vi "test Get Array Size.vi"(8 "error in (no error)":errorcluster, 11 "TestCase in":refnum<class "Python String Parsing Utility Tests.lvclass">) -> (0 "error out":errorcluster, 3 "TestCase out":refnum<class "Python String Parsing Utility Tests.lvclass">)   [LabVIEW 2020, in "Python String Parsing Utility Tests.lvclass"]
uses:
  Python String Parsing Utility Tests.lvclass
  Python String Parsing Utility Tests.lvclass/Python String Parsing Utility Tests.ctl
  <vilib>/addons/_JKI Toolkits/VI Tester/TestCase.llb/TestCase.lvclass
  source/jki_python_data_tools.lvlib
  C:/Program Files/National Instruments/LabVIEW 2020/vi.lib/addons/_JKI Toolkits/VI Tester/TestCase.llb/TestCase.lvclass
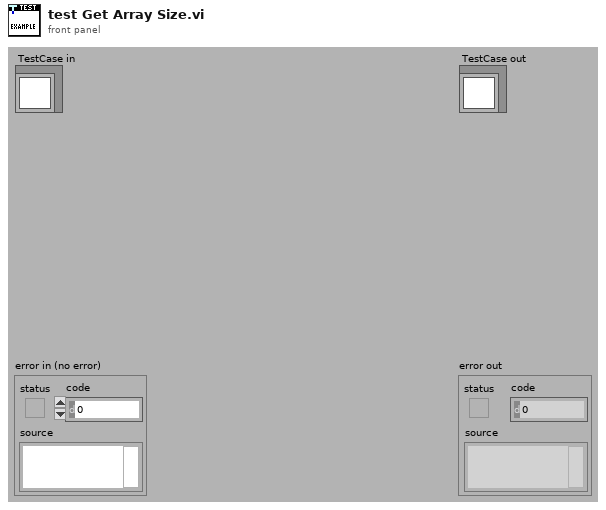
[diagram p1: front panel]
types:
  T1 = cluster{"Input":string, "Expected Result":i32, "Comment":string}[]
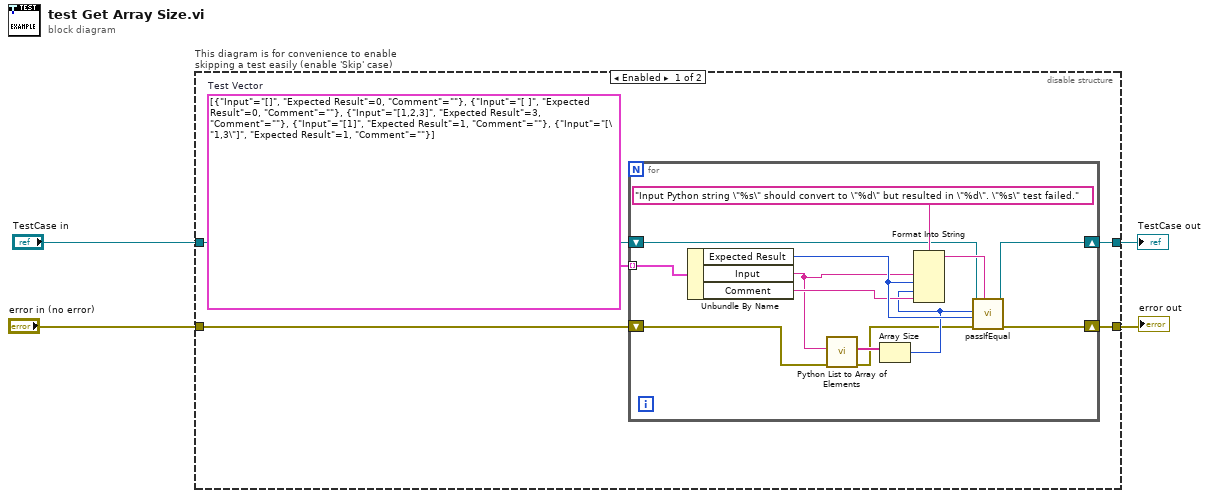
[diagram p0: block diagram]
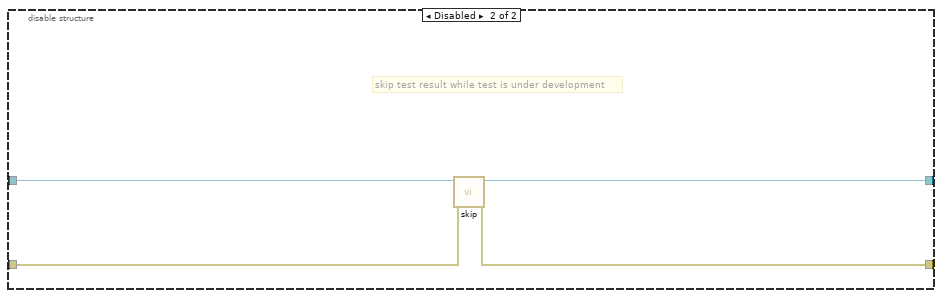
[diagram p2: hidden frame]
diagram:
  n1 = disable-structure "This diagram is for convenience to enable skipping a test easily (enable 'Skip' case)" shown="Enabled" {
    disable-tunnel: "TestCase in" -> [w8 w26]
    disable-tunnel: [w6 w24] -> w1
    disable-tunnel: [w5 w25] -> w3
    disable-tunnel: "error in (no error)" -> [w7 w23]
    frame Enabled {
      w9 = T1 [{"Input"="[]", "Expected Result"=0, "Comment"=""}, {"Input"="[ ]", "Expected Result"=0, "Comment"=""}, {"Input"="[1,2,3]", "Expected Result"=3, "Comment"=""}, {"Input"="[1]", "Expected Result"=1, "Comment"=""}, {"Input"="[\"1,3\"]", "Expected Result"=1, "Comment"=""}]  # Test Vector
      n2 = for {
        tunnel: w9 -> [w10] mode=indexing
        shift-right: [w22] -> w5
        shift-left: w7 -> [w12]
        shift-right: [w18] -> w6
        shift-left: w8 -> [w19]
        n3 = Unbundle By Name(w10) -> ("Expected Result"=w17:i32, "Input"=w13:string, "Comment"=w16:string)
        n4 = call "Python List to Array of Elements.vi"("error in (no error)"=w12, "Python List"=w13) -> ("error out"=w11:errorcluster, "Elements"=w15:string[])  [unwired: 8 in]
        n5 = Array Size(array=w15) -> (size(s)=w14:i32)
        n6 = Format Into String(format string="Input Python string \"%s\" should convert to \"%d\" but resulted in \"%d\". \"%s\" test failed.", w13, w17, w14, w16) -> (resulting string=w21:string)  [unwired: 2 in, 1 out]
        n7 = call-dynamic "passIfEqual.vi"("custom report message (\"\")"=w21, "error in (no error)"=w11, "y"=w17, "x"=w14, "TestCase in"=w19) -> ("error out"=w22:errorcluster, "TestCase out"=w18:refnum<class "Python String Parsing Utility Tests.lvclass">)  [unwired: 5 in]
      }
    }
    frame Disabled {
      # "skip test result while test is under development"
      n8 = call <vilib>:"skip.vi"("error in (no error)"=w23, "TestCase in"=w26) -> ("error out"=w25:errorcluster, "TestCase out"=w24:refnum<class "Python String Parsing Utility Tests.lvclass">)  [unwired: 8 in]
    }
  }
  "error out" <- w3
  "TestCase out" <- w1
